vi "Periodic Tasks.vi"(8 "error in":errorcluster) -> ()   [LabVIEW 2014]
doc: "This VI runs in parallel to other tasks. It can contain as many user-defined periodic loops as you need. These can carry out PID or other sorts of timed response."
uses:
  <vilib>/Rock Robotics/Network Tables/SD Read Number.vi
panel:
  out "LIDAR Data":cluster{"magnitude":dbl, "phase":dbl}[](array[cluster])
  in  "Take Scan":bool
  in  "Save Scan As":dbl
  out "Saved Data":cluster{"magnitude":dbl, "phase":dbl}[][](array[cluster])
  out "Live Scan":picture
  in  "Saved":T1={"maximum"=500.0, "minimum"=0.0, "clip to min"=FALSE, "log?(F)"=FALSE, "grid color"=6710886, "plot color"=16711680, "fmt and prec"={"format"=enum."Decimal", "precision"=0}, "visible section"=8}
  out "Saved Scan":picture
  in  "Live":T1={"maximum"=500.0, "minimum"=0.0, "clip to min"=FALSE, "log?(F)"=FALSE, "grid color"=6710886, "plot color"=16711680, "fmt and prec"={"format"=enum."Decimal", "precision"=0}, "visible section"=8}
  in  "Display Scan":dbl
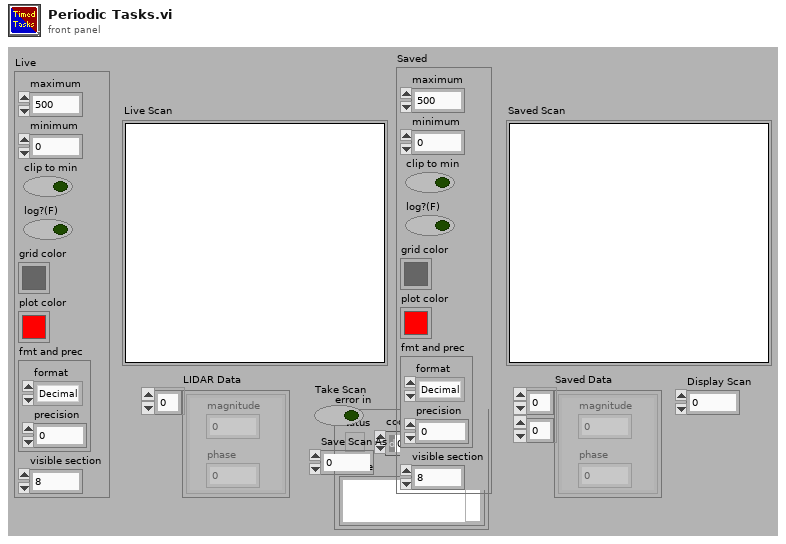
[diagram p1: front panel]
types:
  T1 = cluster{"maximum":dbl, "minimum":dbl, "clip to min":bool, "log?(F)":bool, "grid color":u32, "plot color":u32, "fmt and prec":cluster{"format":enum8{"Decimal", "Scientific", "Engineering", "Binary", "Octal", "Hex"}, "precision":u8}, "visible section":u16}
  T2 = typedef "LVBoundsTypeDef.ctl" = cluster{"Width":u32, "Height":u32}
  T3 = cluster{"[0]":i32, "[1]":i32, "[2]":i32, "[3]":i32, "[4]":i32, "[5]":i32, "[6]":i32, "[7]":i32, "[8]":i32}
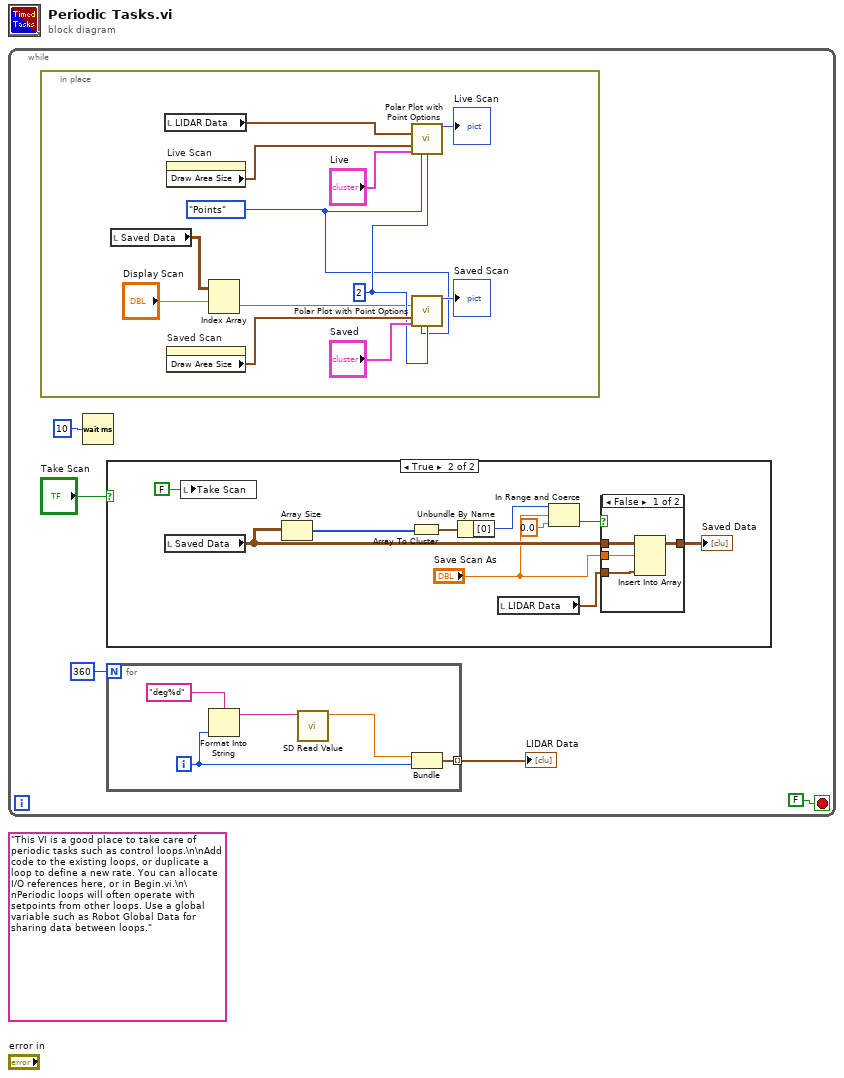
[diagram p0: block diagram]
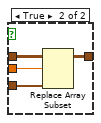
[diagram p3: hidden frame]
diagram:
  (unwired) "This VI is a good place to take care of periodic tasks such as control loops.\n\nAdd code to the existing loops, or duplicate a loop to define a new rate. You can allocate I/O references here, or in Begin.vi.\n\nPeriodic loops will often operate with setpoints from other loops. Use a global variable such as Robot Global Data for sharing data between loops."
  n1 = while {
    stop <- FALSE stop-if-true
    n2 = in-place {
      w10 = 2
      w9 = enum16{"Lines", "Points"}."Points" ("Lines/Points")
      n3 = local read "Saved Data"() -> (w8:cluster{"magnitude":dbl, "phase":dbl}[][])
      n4 = local read "LIDAR Data"() -> (w15:cluster{"magnitude":dbl, "phase":dbl}[])
      n5 = property on="Live Scan" class="Pict"() -> ("Draw Area Size"=w16:T2)  [unwired: 2 in, 2 out]
      n6 = property on="Saved Scan" class="Pict"() -> ("Draw Area Size"=w14:T2)  [unwired: 2 in, 2 out]
      n7 = Index Array(array=w8, index (row)="Display Scan") -> (element=w6:cluster{"magnitude":dbl, "phase":dbl}[])  [unwired: 1 in]
      n8 = call <vilib>:"Polar Plot with Point Options.vi"("data array [mag, phase (deg)]"=w15, "dimensions (w,h)"=w16, "polar attributes"="Live", "Lines/Points"=w9, "Size"=w10) -> ("new picture"=→"Live Scan":picture)  [unwired: 10 in]
      n9 = call <vilib>:"Polar Plot with Point Options.vi"("data array [mag, phase (deg)]"=w6, "dimensions (w,h)"=w14, "polar attributes"="Saved", "Lines/Points"=w9, "Size"=w10) -> ("new picture"=→"Saved Scan":picture)  [unwired: 10 in]
    }
    n10 = Wait (ms)(milliseconds to wait=u32 10) -> ()  [unwired: 1 out]
    n11 = case shown="True" "Take Scan" {
      frame False {
      }
      frame True {
        n12 = local read "Saved Data"() -> (w20:cluster{"magnitude":dbl, "phase":dbl}[][])
        n13 = local write "Take Scan"(FALSE) -> ()
        n14 = Array Size(array=w20) -> (size(s)=w26:i32[])
        n15 = Array To Cluster(array=w26) -> (cluster=w25:T3)
        n16 = Unbundle By Name(w25) -> ("[0]"=w24:i32)
        n17 = local read "LIDAR Data"() -> (w21:cluster{"magnitude":dbl, "phase":dbl}[])
        n18 = In Range and Coerce(upper limit=w24, x="Save Scan As", lower limit=0.0) -> (In Range?=w23:bool)  [unwired: 1 out]
        n19 = case shown="False" w23 {
          tunnel: w21 -> [w29 w35]
          tunnel: w20 -> [w30 w34]
          tunnel: "Save Scan As" -> [w31 w33]
          tunnel: [w28 w32] -> w18
          frame False {
            n20 = Insert Into Array(array=w30, index (row)=w31, new element=w29) -> (w28:cluster{"magnitude":dbl, "phase":dbl}[][])  [unwired: 1 in]
          }
          frame True {
            n21 = Replace Array Subset(array=w34, new element=w35, index (row)=w33) -> (w32:cluster{"magnitude":dbl, "phase":dbl}[][])  [unwired: 1 in]
          }
        }
        "Saved Data" <- w18
      }
    }
    n22 = for {
      N: 360 -> [_]
      tunnel: [w36] -> w2 mode=indexing
      i -> [w37]
      n23 = Format Into String(format string="deg%d", w37) -> (resulting string=w39:string)  [unwired: 2 in, 1 out]
      n24 = call-poly <vilib>:"SD Read Value.vi"("Name"=w39) -> ("Numeric"=w38:dbl)  [unwired: 8 in, 2 out]
      n25 = Bundle("Numeric"=w38, w37) -> (w36:cluster{"Numeric":dbl, i32})  [unwired: 1 in]
    }
    "LIDAR Data" <- w2
  }
